vi "tsapp_configure_canfd_regs.vi"() -> ()   [LabVIEW 2019]
panel:
  in  "簇":T1
  out "路径输出":path
  in  "路径输入":path
  out "返回类型":i32
  # "lfdmNormal = 0, lfdmACKOff = 1, lfdmRestricted = 2, lfdmInternalLoopback = 3, lfdmExternalLoopback = 4"
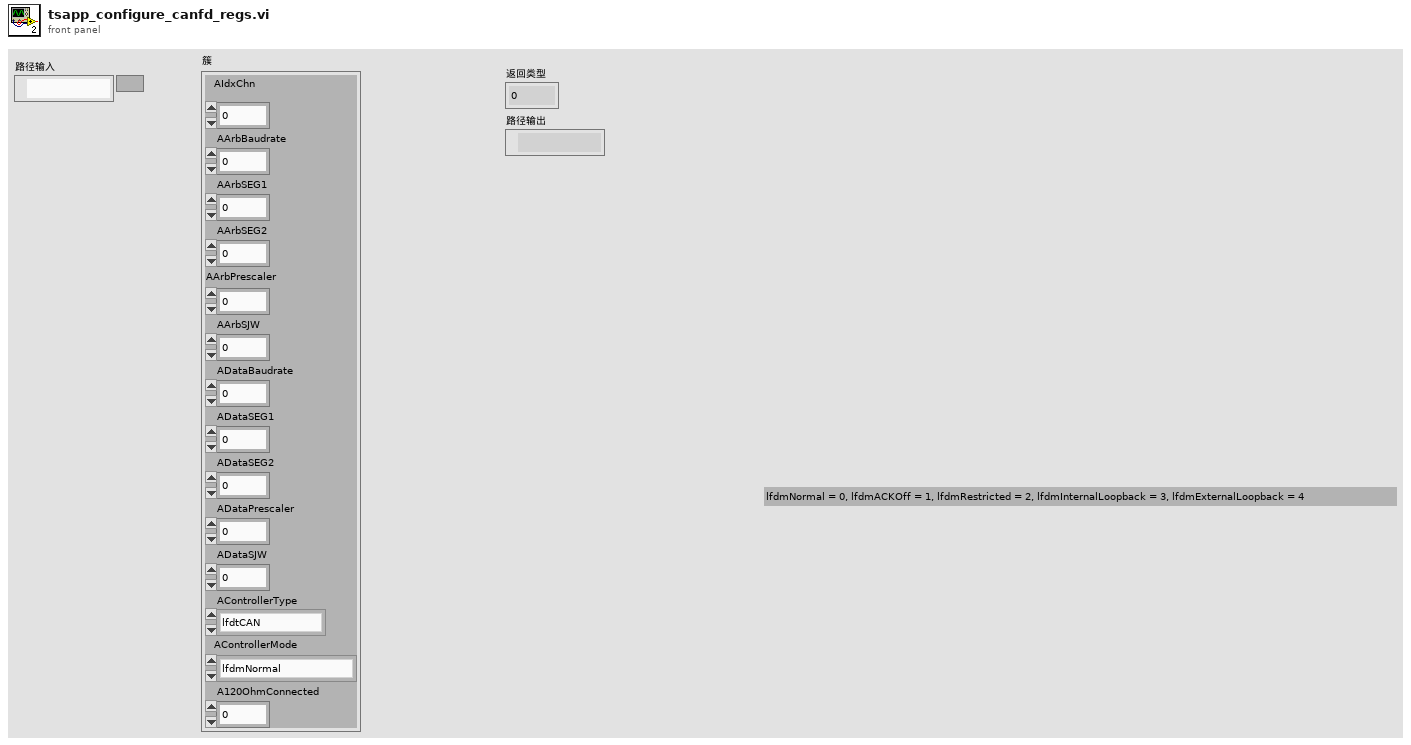
[diagram p1: front panel]
types:
  T1 = cluster{"AIdxChn":i32, "AArbBaudrate":sgl, "AArbSEG1":i32, "AArbSEG2":i32, "AArbPrescaler":i32, "AArbSJW":i32, "ADataBaudrate":sgl, "ADataSEG1":i32, "ADataSEG2":i32, "ADataPrescaler":i32, "ADataSJW":i32, "AControllerType":enum32{"lfdtCAN", "lfdtISOCAN", "lfdtNonISOCAN"}, "AControllerMode":enum32{"lfdmNormal", "lfdmACKOff", "lfdmRestricted", "lfdmInternalLoopback", "lfdmExternalLoopback"}, "A120OhmConnected":i32}
  T2 = enum32{"lfdmNormal", "lfdmACKOff", "lfdmRestricted", "lfdmInternalLoopback", "lfdmExternalLoopback"}
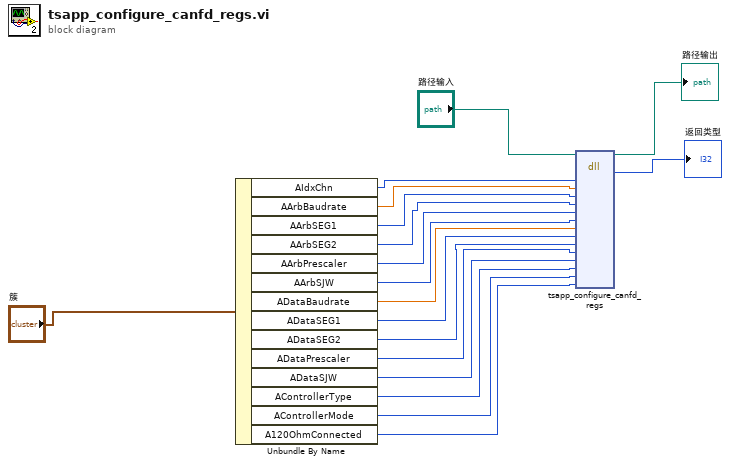
[diagram p0: block diagram]
diagram:
  n1 = Unbundle By Name("簇") -> ("AIdxChn"=w14:i32, "AArbBaudrate"=w13:sgl, "AArbSEG1"=w12:i32, "AArbSEG2"=w11:i32, "AArbPrescaler"=w10:i32, "AArbSJW"=w9:i32, "ADataBaudrate"=w8:sgl, "ADataSEG1"=w7:i32, "ADataSEG2"=w6:i32, "ADataPrescaler"=w5:i32, "ADataSJW"=w4:i32, "AControllerType"=w3:enum32{"lfdtCAN", "lfdtISOCAN", "lfdtNonISOCAN"}, "AControllerMode"=w2:T2, "A120OhmConnected"=w1:i32)
  n2 = dll-call lib="C:/Users/XYY/Desktop/LabView Demo/TSCAN_LB2018_V1.3_20220301/Config/TSMaster.dll" fn="tsapp_configure_canfd_regs"(path in="路径输入", "AIdxChn"=w14, "AArbBaudrate"=w13, "AArbSEG1"=w12, "AArbSEG2"=w11, "AArbPrescaler"=w10, "AArbSJW"=w9, "ADataBaudrate"=w8, "ADataSEG1"=w7, "ADataSEG2"=w6, "ADataPrescaler"=w5, "ADataSJW"=w4, "AControllerType"=w3, "AControllerMode"=w2, "A120OhmConnected"=w1) -> (path out=→"路径输出":path, "返回类型"=→"返回类型":i32)  [unwired: 16 in, 1 out]
